vi "Connection (global).vi"(0 "PC Connected In":bool, 2 "Mode":enum16{"Read", "Write"}(ring)) -> (4 "PC Connected Out":bool)   [LabVIEW 2013]
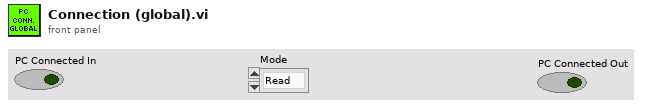
[diagram p1: front panel]
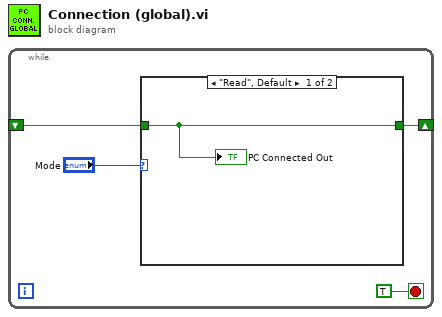
[diagram p0: block diagram]
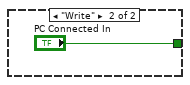
[diagram p2: hidden frame]
diagram:
  n1 = while {
    shift-right: [w2] -> _
    shift-left: _ -> [w1]
    stop <- TRUE stop-if-true
    n2 = case shown="\"Read\", Default" "Mode" {
      tunnel: [w5 "PC Connected In"] -> w2
      tunnel: w1 -> [w5 _]
      frame "Read", Default {
        "PC Connected Out" <- w5
      }
      frame "Write" {
      }
    }
  }
